vi "Read Bar Code.vi"(6 "error in (no error)":errorcluster) -> (0 "error out":errorcluster, 2 "concatenated string":string, 3 "bar code read":string)   [LabVIEW 2018]
panel:
  in  "stop":bool
  in  "bar code":string
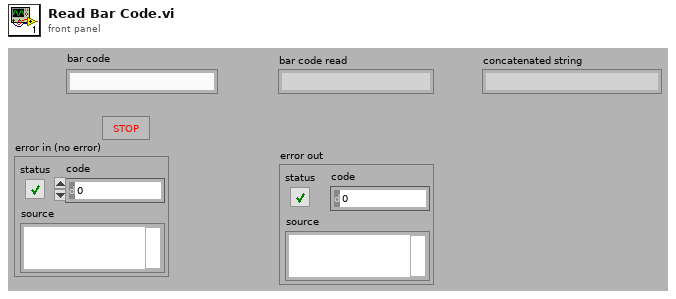
[diagram p1: front panel]
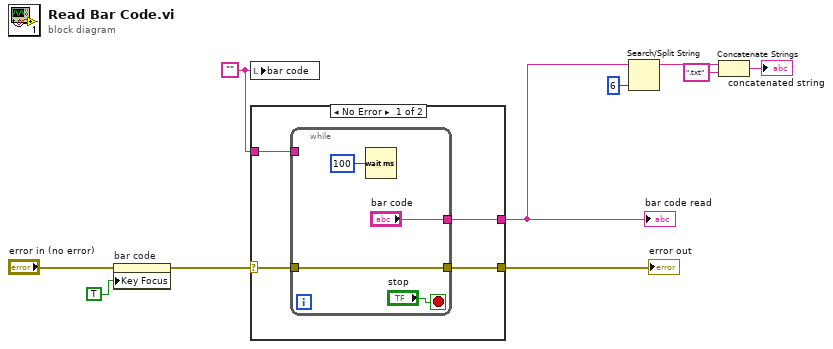
[diagram p0: block diagram]
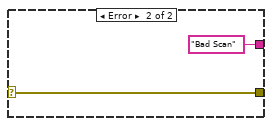
[diagram p2: hidden frame]
diagram:
  w8 = ""
  n1 = property on="bar code" class="Str"(error in="error in (no error)", "Key Focus"=TRUE) -> (error out=w9:errorcluster)  [unwired: 1 in, 1 out]
  n2 = local write "bar code"(w8) -> ()
  n3 = case shown="No Error" w9 {
    selector: w9 -> [w13 w20]
    tunnel: [w14 "Bad Scan" ("bar code")] -> w5
    tunnel: w8 -> [w12 _]
    tunnel: [w11 w20] -> w6
    frame No Error {
      n4 = while {
        tunnel: ["bar code"] -> w14
        tunnel: w13 -> [w15]
        tunnel: w12 -> [_]
        tunnel: [w15] -> w11
        stop <- "stop" stop-if-true
        n5 = Wait (ms)(milliseconds to wait=u32 100) -> ()  [unwired: 1 out]
      }
    }
    frame Error {
    }
  }
  "bar code read" <- w5
  "error out" <- w6
  n6 = Search/Split String(string=w5, offset (0)=6) -> (substring before match=w3:string)  [unwired: 1 in, 2 out]
  n7 = Concatenate Strings(w3, ".txt" ("string")) -> (→"concatenated string":string)
